vi "TurnSmooth.vi"(4 "Pivot":bool, 5 "Min Power":dbl, 6 "FirstTime?":bool, 7 "Target Range":dbl, 8 "Current Position":dbl, 9 "Dir&Deg":dbl, 10 "Slow Range":dbl, 11 "Motor Power In":dbl) -> (0 "Done":bool, 1 "DegToTarget":dbl, 2 "Right Motor Power":dbl, 3 "Left Motor Power":dbl)   [LabVIEW 2017]
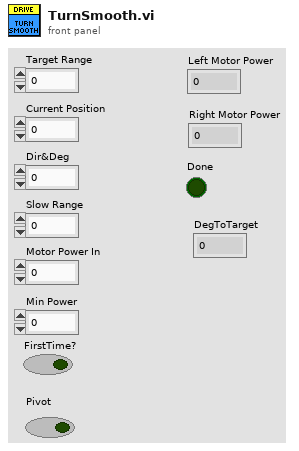
[diagram p1: front panel]
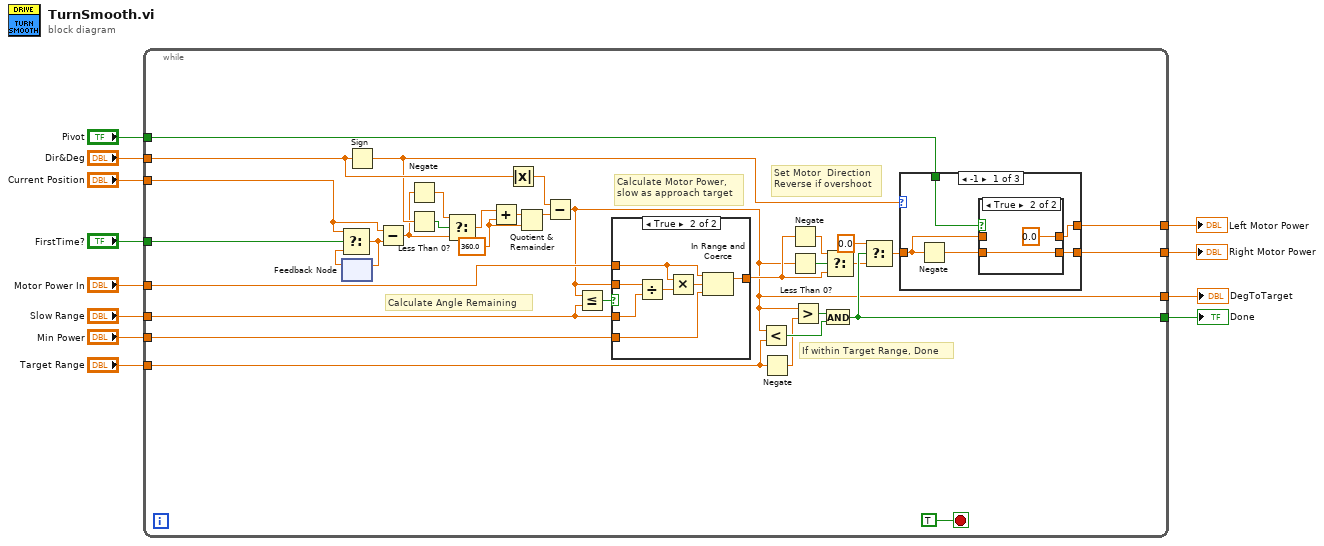
[diagram p0: block diagram]
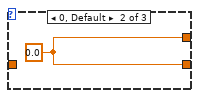
[diagram p3: hidden frame]
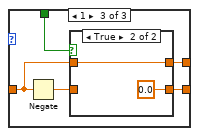
[diagram p4: hidden frame]
diagram:
  n1 = while {
    tunnel: "Slow Range" -> [w46]
    tunnel: "Min Power" -> [w45]
    tunnel: "Motor Power In" -> [w44]
    tunnel: "Dir&Deg" -> [w40]
    tunnel: "Current Position" -> [w41]
    tunnel: [w43] -> w2
    tunnel: [w15] -> w3
    tunnel: [w37] -> w7
    tunnel: "FirstTime?" -> [w42]
    tunnel: "Target Range" -> [w38]
    tunnel: "Pivot" -> [w14]
    tunnel: [w13] -> w1
    stop <- TRUE stop-if-true
    w27 = 360.0 ("value")
    # "If within Target Range, Done"
    # "Calculate Angle Remaining"
    # "Calculate Motor Power,\nslow as approach target"
    # "Set Motor  Direction\nReverse if overshoot"
    n2 = feedback #1() -> (w35:dbl)  [unwired: 1 in]
    n3 = Select(t=w41, s=w42, f=w35) -> (s? t:f=w34:dbl)
    n4 = feedback-in #1(w34) -> ()
    n5 = Sign(1:w40) -> (0:w31:dbl)
    n6 = Subtract(x=w41, y=w34) -> (x-y=w29:dbl)
    n7 = Negate(x=w29) -> (-x=w30:dbl)
    n8 = Less Than 0?(x=w31) -> (x < 0?=w32:bool)
    n9 = Select(t=w30, s=w32, f=w29) -> (s? t:f=w28:dbl)
    n10 = Add(x=w28, y=w27) -> (x+y=w33:dbl)
    n11 = Absolute Value(x=w40) -> (abs(x)=w25:dbl)
    n12 = Quotient & Remainder(x=w33, y=w27) -> (x-y*floor(x/y)=w26:dbl)  [unwired: 1 out]
    n13 = Subtract(x=w25, y=w26) -> (x-y=w13:dbl)
    n14 = Less Or Equal?(x=w13, y=w46) -> (x <= y?=w36:bool)
    n15 = case shown="True" w36 {
      tunnel: [w66 w73] -> w17
      tunnel: w44 -> [w66 w72]
      tunnel: w45 -> [_ w71]
      tunnel: w46 -> [_ w70]
      tunnel: w13 -> [_ w67]
      frame False {
      }
      frame True {
        n16 = Divide(x=w67, y=w70) -> (x/y=w68:dbl)
        n17 = Multiply(x=w72, y=w68) -> (x*y=w69:dbl)
        n18 = In Range and Coerce(upper limit=w72, x=w69, lower limit=w71) -> (coerced(x)=w73:dbl)  [unwired: 1 out]
      }
    }
    n19 = Less?(x=w13, y=w38) -> (x < y?=w24:bool)
    n20 = Negate(x=w38) -> (-x=w23:dbl)
    n21 = Negate(x=w17) -> (-x=w20:dbl)
    n22 = Less Than 0?(x=w13) -> (x < 0?=w21:bool)
    n23 = Greater?(x=w13, y=w23) -> (0:w22:bool)
    n24 = And(x=w22, y=w24) -> (x .and. y?=w37:bool)
    n25 = Select(t=w20, s=w21, f=w17) -> (s? t:f=w19:dbl)
    n26 = Select(t=0.0, s=w37, f=w19) -> (s? t:f=w16:dbl)
    n27 = case shown="-1" w31 {
      tunnel: [w49 w56 w60] -> w15
      tunnel: [w47 w56 w59] -> w43
      tunnel: w16 -> [w48 _ w58]
      tunnel: w14 -> [w51 _ w57]
      frame -1 {
        n28 = Negate(x=w48) -> (-x=w50:dbl)
        n29 = case shown="True" w51 {
          tunnel: w50 -> [w53 w54]
          tunnel: [w53 w54] -> w49
          tunnel: w48 -> [w52 _]
          tunnel: [w52 0.0] -> w47
          frame False {
          }
          frame True {
          }
        }
      }
      frame 0, Default {
        w56 = 0.0
      }
      frame 1 {
        n30 = Negate(x=w58) -> (-x=w61:dbl)
        n31 = case shown="True" w57 {
          tunnel: w61 -> [w63 _]
          tunnel: [w63 0.0] -> w60
          tunnel: [w62 w64] -> w59
          tunnel: w58 -> [w62 w64]
          frame False {
          }
          frame True {
          }
        }
      }
    }
  }
  "Left Motor Power" <- w2
  "Done" <- w7
  "Right Motor Power" <- w3
  "DegToTarget" <- w1
